vi "Start data stream (S).vi"(0 "VISA resource name in":refnum<visa-resource-name>, 3 "Error In":errorcluster) -> (7 "VISA resource name out":refnum<visa-resource-name>, 10 "Error out":errorcluster)   [LabVIEW 2015]
uses:
  Ctls/Cmd str.ctl
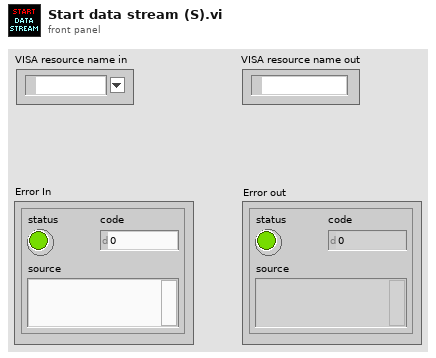
[diagram p1: front panel]
types:
  T1 = typedef "Cmd str.ctl" = string
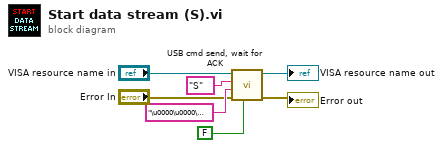
[diagram p0: block diagram]
diagram:
  n1 = call "USB cmd send, wait for ACK.vi"("Wait for ACK?"=FALSE, "Error In"="Error In", "4 byte config str"="\u0000\u0000\u0000\u0000", "Cmd"=T1 "S", "VISA resource name in"="VISA resource name in") -> ("Error out"=→"Error out":errorcluster, "VISA resource name out"=→"VISA resource name out":refnum<visa-resource-name>)  [unwired: 1 in, 2 out]
